vi "Measure Channel Power.vi"(8 "error in":errorcluster, 10 "Channel":T1, 11 "2936r in":refnum<class "2936r.lvclass">) -> (0 "error out":errorcluster, 2 "Power":dbl, 3 "2936r out":refnum<class "2936r.lvclass">)   [LabVIEW 2018, in "2936r.lvlib" / "2936r.lvclass"]
uses:
  2936r.lvclass
  PPLs/Optical Power Meter/Optical Power Meter.lvlibp/Custom Controls/Channel List.ctl
  2936r.lvclass/2936r.ctl
  PPLs/Optical Power Meter/Optical Power Meter.lvlibp
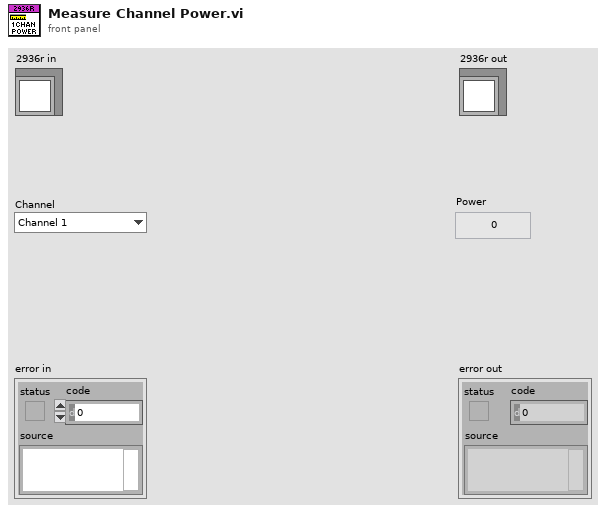
[diagram p1: front panel]
types:
  T1 = typedef "Optical Power Meter.lvlibp/Channel List.ctl" = enum16{"Channel 1", "Channel 2", "Channel 3", "Channel 4"}
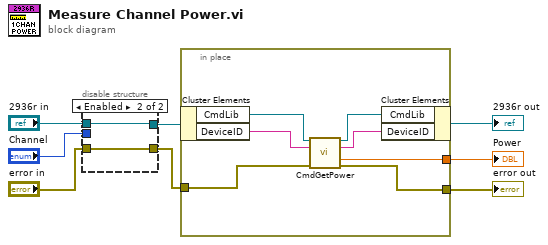
[diagram p0: block diagram]
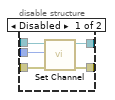
[diagram p2: hidden frame]
diagram:
  n1 = disable-structure shown="Enabled" {
    disable-tunnel: "2936r in" -> [w13 w15]
    disable-tunnel: [w12 w15] -> w4
    disable-tunnel: "error in" -> [w11 w14]
    disable-tunnel: [w10 w14] -> w2
    disable-tunnel: "Channel" -> [w9 _]
    frame Disabled {
      n2 = call-dynamic "Set Channel.vi"("error in (no error)"=w11, "Channel"=w9, "2936r in"=w13) -> ("error out"=w10:errorcluster, "2936r out"=w12:refnum<class "2936r.lvclass">)  [unwired: 7 in]
    }
    frame Enabled {
    }
  }
  n3 = in-place {
    in-place-border: [w18] -> w7
    in-place-border: [w17] -> w6
    in-place-border: w2 -> [w16]
    n4 = in-place-cluster #1(w4) -> ("CmdLib"=w22:refnum<k24>, "DeviceID"=w20:string)
    n5 = call <instrlib>:"CmdGetPower.vi"("PM Cmds In"=w22, "Device Key In"=w20, "error in"=w16) -> ("PM Cmds Out"=w21:refnum<k24>, "Device Key Out"=w19:string, "Power Value"=w18:sgl, "error out"=w17:errorcluster)  [unwired: 8 in, 1 out]
    n6 = in-place-cluster #1("CmdLib"=w21, "DeviceID"=w19) -> (→"2936r out":refnum<class "2936r.lvclass">)
  }
  "error out" <- w6
  "Power" <- w7
